vi "ResizeImage.vi"(8 "error in (no error)":errorcluster, 10 "Image Data":T1, 11 "2D Picture Ref":refnum<vi>) -> (0 "error out":errorcluster, 2 "Image Data (dup)":T1, 3 "Zoomed Picture Ref":refnum<vi>)   [LabVIEW 2017, in "Slide.lvclass"]
uses:
  Slide.lvclass
  <vilib>/picture/picture.llb/imagedata.ctl
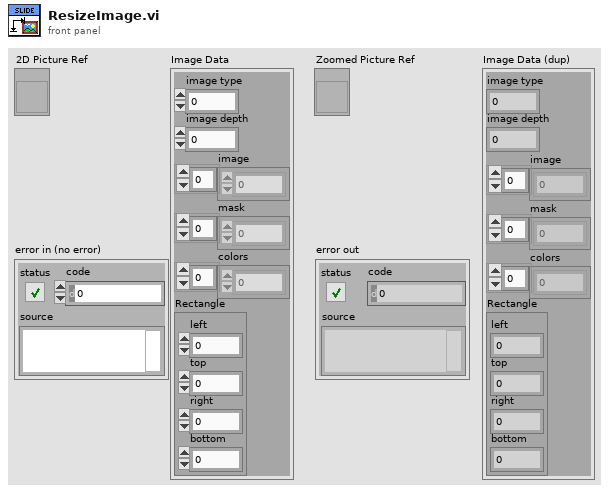
[diagram p1: front panel]
types:
  T1 = typedef "imagedata.ctl" = cluster{"image type":i32, "image depth":i32, "image":u8[], "mask":u8[], "colors":u32[], "Rectangle":cluster{"left":i16, "top":i16, "right":i16, "bottom":i16}}
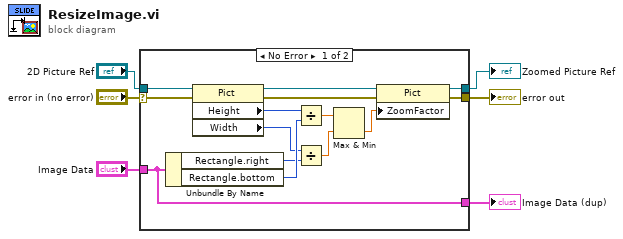
[diagram p0: block diagram]
diagram:
  n1 = case shown="No Error" "error in (no error)" {
    selector: "error in (no error)" -> [w19 w23]
    tunnel: "2D Picture Ref" -> [w20 w21]
    tunnel: [w8 w23] -> w4
    tunnel: "Image Data" -> [w9 w22]
    tunnel: [w9 w22] -> w1
    tunnel: [w7 w21] -> w2
    frame No Error {
      n2 = Unbundle By Name(w9) -> ("Rectangle.right"=w15:i16, "Rectangle.bottom"=w17:i16)
      n3 = property class="Pict"(reference=w20, error in=w19) -> (reference out=w11:refnum<vi>, error out=w10:errorcluster, "Height"=w18:u32, "Width"=w16:u32)
      n4 = Divide(x=w18, y=w17) -> (x/y=w14:dbl)
      n5 = Divide(x=w16, y=w15) -> (x/y=w13:dbl)
      n6 = Max & Min(x=w14, y=w13) -> (min(x,y)=w12:dbl)  [unwired: 1 out]
      n7 = property class="Pict"(reference=w11, error in=w10, "ZoomFactor"=w12) -> (reference out=w7:refnum<vi>, error out=w8:errorcluster)
    }
    frame Error {
    }
  }
  "error out" <- w4
  "Zoomed Picture Ref" <- w2
  "Image Data (dup)" <- w1
